vi "setvcan3setting.vi"(8 "error in (no error)":errorcluster, 10 "SVCAN3Setting":T1, 11 "hObject":i32) -> (0 "error out":errorcluster, 3 "hObject Out":i32)   [LabVIEW 2009]
doc: "this vi applys the SVCAN3Settings to the device\n\n12/21/2010 1.0.0 jyg\n- initial release"
uses:
  ctl svcansetting.ctl
  NEO VI Example/data/icsneo40.dll
panel:
  in  "Save Setting Permanently? (F)":bool
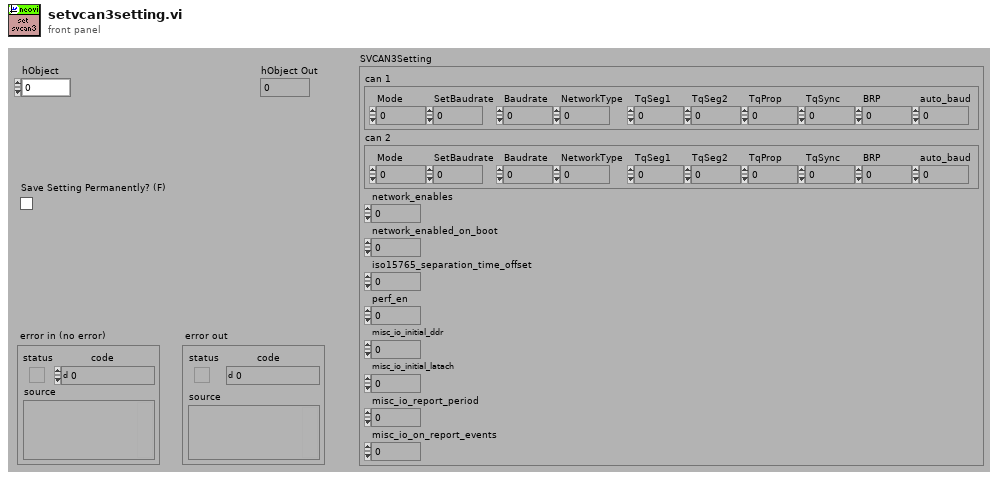
[diagram p1: front panel]
types:
  T1 = typedef "ctl SVCANSetting.ctl" = cluster{"can 1":cluster{"Mode":u8, "SetBaudrate":u8, "Baudrate":u8, "NetworkType":u8, "TqSeg1":u8, "TqSeg2":u8, "TqProp":u8, "TqSync":u8, "BRP":u16, "auto_baud":u16}, "can 2":cluster{"Mode":u8, "SetBaudrate":u8, "Baudrate":u8, "NetworkType":u8, "TqSeg1":u8, "TqSeg2":u8, "TqProp":u8, "TqSync":u8, "BRP":u16, "auto_baud":u16}, "network_enables":u16, "network_enabled_on_boot":u16, "iso15765_separation_time_offset":i16, "perf_en":u16, "misc_io_initial_ddr":u16, "misc_io_initial_latach":u16, "misc_io_report_period":u16, "misc_io_on_report_events":u16}
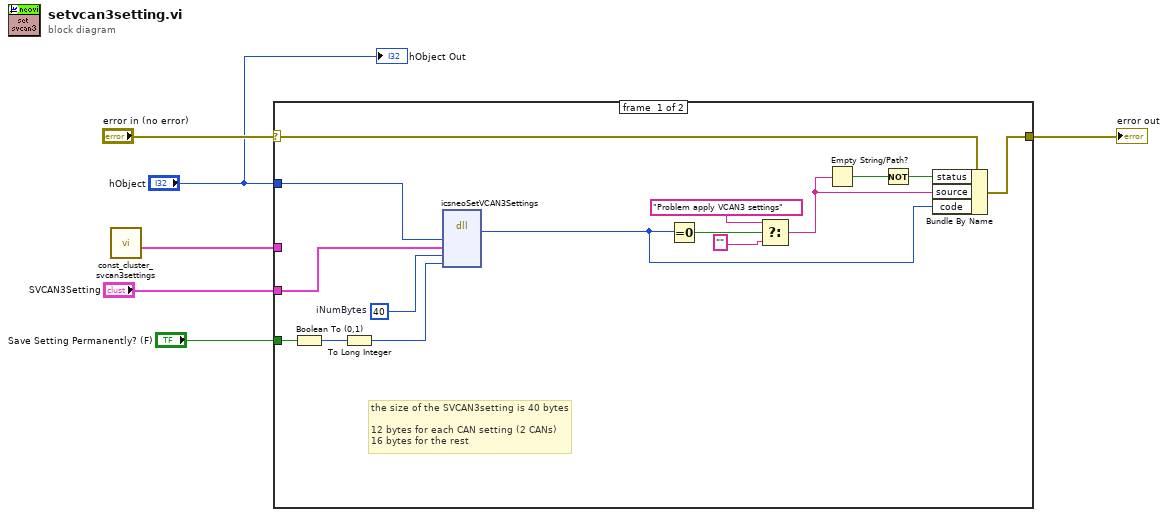
[diagram p0: block diagram]
diagram:
  n1 = call "const_cluster_svcan3settings.vi"() -> ("SVCAN3Settings"=w3:T1)
  n2 = case shown="No Error" "error in (no error)" {
    selector: "error in (no error)" -> [w17 w22]
    tunnel: "hObject" -> [w12 _]
    tunnel: [w18 w22] -> w6
    tunnel: w3 -> [_ _]
    tunnel: "SVCAN3Setting" -> [w10 _]
    tunnel: "Save Setting Permanently? (F)" -> [w9 _]
    frame #0 {
      w11 = 40  # iNumBytes
      # "the size of the SVCAN3setting is 40 bytes\n\n12 bytes for each CAN setting (2 CANs)\n16 bytes for the rest"
      n3 = Boolean To (0,1)(Boolean=w9) -> (0, 1=w8:i16)
      n4 = To Long Integer(number=w8) -> (32bit integer=w7:i32)
      n5 = dll-call lib="C:/WINDOWS/system32/icsneo40.dll" fn="icsneoSetVCAN3Settings"("hObject"=w12, "SVCAN3Setting"=w10, "iNumBytes"=w11, "bSaveToEEPROM"=w7) -> ("return type"=w16:i32)  [unwired: 7 in, 2 out]
      n6 = Equal To 0?(x=w16) -> (x = 0?=w15:bool)
      n7 = Select(t="Problem apply VCAN3 settings", s=w15, f="") -> (s? t:f=w14:string)
      n8 = Empty String/Path?(string/path=w14) -> (empty?=w20:bool)
      n9 = Not(x=w20) -> (.not. x?=w19:bool)
      n10 = Bundle By Name(cluster=w17, "status"=w19, "source"=w14, "code"=w16) -> (w18:errorcluster)
    }
    frame #1 {
    }
  }
  "error out" <- w6
  "hObject Out" <- "hObject"
